vi "Check Data Size (excel).vi"(1 "error in (no error)":errorcluster, 2 "rect":T1, 3 "depth":u8, 4 "flattened image data":u8[](array[numeric])) -> (0 "error out":errorcluster)   [LabVIEW 2020, in "NI_ReportGenerationToolkit.lvlib"]
doc: "Checks the flattened data to see if the size of the data in bytes is what we expect it to be based on its bounds and depth."
uses:
  <vilib>/addons/_office/NI_ReportGenerationToolkit.lvlib
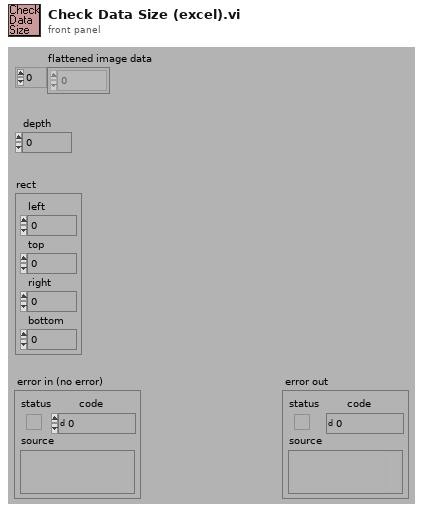
[diagram p1: front panel]
types:
  T1 = cluster{"left":i16, "top":i16, "right":i16, "bottom":i16}
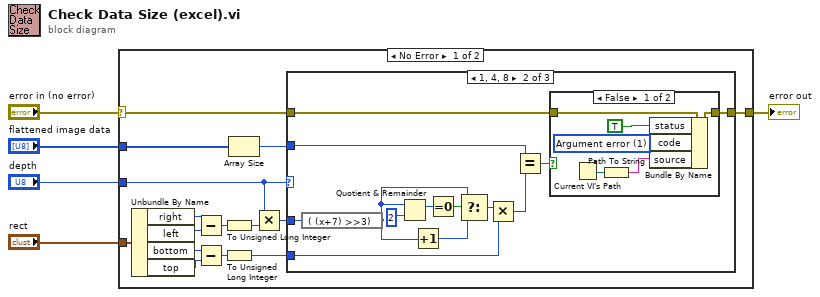
[diagram p0: block diagram]
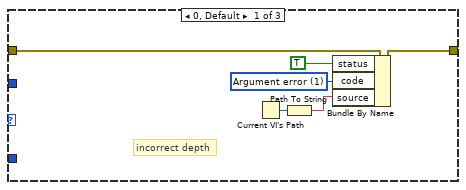
[diagram p2: hidden frame]
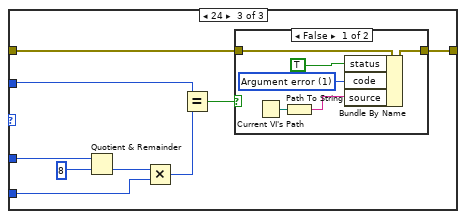
[diagram p4: hidden frame]
diagram:
  n1 = case shown="No Error" "error in (no error)" {
    selector: "error in (no error)" -> [w6 w63]
    tunnel: "depth" -> [w17 _]
    tunnel: "rect" -> [w16 _]
    tunnel: [w10 w63] -> w3
    tunnel: "flattened image data" -> [w9 _]
    frame No Error {
      n2 = Unbundle By Name(w16) -> ("right"=w11:i16, "left"=w12:i16, "bottom"=w15:i16, "top"=w14:i16)
      n3 = Subtract(x=w11, y=w12) -> (x-y=w13:i16)
      n4 = Subtract(x=w15, y=w14) -> (x-y=w18:i16)
      n5 = To Unsigned Long Integer(number=w13) -> (unsigned 32bit integer=w8:u32)
      n6 = To Unsigned Long Integer(number=w18) -> (unsigned 32bit integer=w7:u32)
      n7 = Array Size(array=w9) -> (size(s)=w20:i32)
      n8 = Multiply(x=w17, y=w8) -> (x*y=w19:u32)
      n9 = case shown="1, 4, 8" w17 {
        tunnel: w6 -> [w22 w33 w53]
        tunnel: [w21 w37 w52] -> w10
        tunnel: w7 -> [_ w36 w48]
        tunnel: w19 -> [_ w35 w51]
        tunnel: w20 -> [_ w34 w55]
        frame 0, Default {
          w25 = 1 items=["No error", "Argument error", "Memory is full", "Out of zone", "End of file", "File already open", "Generic file I/O error", "File not found", "File permission error", "Disk is full", "Duplicate path", "Too many files open", "System feature not enabled", "Resource file not found", "Cannot add resource", "Resource not found", "Image not found", "Image memory error", "Pen does not exist", "Config type invalid", "Config token not found", "Config parse error", "Config memory error", "Bad external code format", "Bad external code offset", "External code not present", "Null window", "Destroy window error", "Null menu", "Print aborted", "Bad print record", "Print driver error", "Windows error during printing", "Memory error during printing", "Print dialog error", "Generic print error", "Invalid device refnum", "Device not found", "Device parameter error", "Device unit error", "Cannot open device", "Device call aborted", "Generic error", "Cancelled by user", "Object ID too low", "Object ID too high", "Object not in heap", "Unknown heap", "Unknown object (invalid DefProc)", "Unknown object (DefProc not in table)", "Message out of range", "Invalid (null) method", "Unknown message", "Manager call not supported", "Bad address", "Network operation in progress", "Network operation timed out", "Connection is busy", "Network attribute not supported", "Network error", "Address in use", "System out of memory", "Connection aborted", "Connection refused", "Not connected", "Already connected", "Connection closed", "Initialization error (interapplication manager)", "Bad occurrence", "Wait on unbound occurrence handler", "Occurrence queue overflow", "Datalog type conflict", "Unused", "Unrecognized type (interapplication manager)", "Memory corrupt", "Failed to make temporary DLL", "Old CIN version", "Drag socket not found", "Failed to load drop-object", "Failed to register OLE object", "Failed to release OLE object", "Format specifier type mismatch", "Unknown format specifier", "Too few format specifiers", "Too many format specifiers", "Scan failed", "Newer CIN version", "Error converting to variant", "Runtime menu error", "Password tampered", "Variant attribute not found", "Incompatible variant data type", "Event data is not available", "Event Store is not present", "Occurrence is not found", "Event Queue is not created", "Event info is not available", "Refnum passed is NULL", "Error retrieving Class GUID", "Error retrieving CoClass GUID", "Error retrieving TypeLib GUID.", "Bad built application magic bytes.", "Specific driver is different from the specific driver associated with the Logical Name.", "There is no session opened to the class driver.", "Max Error", "MAX - Error with config objects", "MAX - Error loading configuration", "MAX - Group not supported"]
          # "incorrect depth"
          n10 = Current VI's Path() -> (path=w24:path)
          n11 = Path To String(path=w24) -> (string=w23:string)
          n12 = Bundle By Name(cluster=w22, "status"=TRUE, "code"=w25, "source"=w23) -> (w21:errorcluster)
        }
        frame 1, 4, 8 {
          n13 = expression code="(\t(x+7) >>3)"(w35) -> (w28:u32)
          n14 = Quotient & Remainder(x=w28, y=u32 2 ("x")) -> (x-y*floor(x/y)=w32:u32)  [unwired: 1 out]
          n15 = Increment(x=w28) -> (x+1=w31:u32)
          n16 = Equal To 0?(x=w32) -> (x = 0?=w30:bool)
          n17 = Select(t=w28, s=w30, f=w31) -> (s? t:f=w29:u32)
          n18 = Multiply(x=w29, y=w36) -> (x*y=w39:u32)
          n19 = Equal?(x=w34, y=w39) -> (x = y?=w38:bool)
          n20 = case shown="False" w38 {
            tunnel: w33 -> [w41 w46]
            tunnel: [w40 w46] -> w37
            frame False {
              w44 = 1 items=["No error", "Argument error", "Memory is full", "Out of zone", "End of file", "File already open", "Generic file I/O error", "File not found", "File permission error", "Disk is full", "Duplicate path", "Too many files open", "System feature not enabled", "Resource file not found", "Cannot add resource", "Resource not found", "Image not found", "Image memory error", "Pen does not exist", "Config type invalid", "Config token not found", "Config parse error", "Config memory error", "Bad external code format", "Bad external code offset", "External code not present", "Null window", "Destroy window error", "Null menu", "Print aborted", "Bad print record", "Print driver error", "Windows error during printing", "Memory error during printing", "Print dialog error", "Generic print error", "Invalid device refnum", "Device not found", "Device parameter error", "Device unit error", "Cannot open device", "Device call aborted", "Generic error", "Cancelled by user", "Object ID too low", "Object ID too high", "Object not in heap", "Unknown heap", "Unknown object (invalid DefProc)", "Unknown object (DefProc not in table)", "Message out of range", "Invalid (null) method", "Unknown message", "Manager call not supported", "Bad address", "Network operation in progress", "Network operation timed out", "Connection is busy", "Network attribute not supported", "Network error", "Address in use", "System out of memory", "Connection aborted", "Connection refused", "Not connected", "Already connected", "Connection closed", "Initialization error (interapplication manager)", "Bad occurrence", "Wait on unbound occurrence handler", "Occurrence queue overflow", "Datalog type conflict", "Unused", "Unrecognized type (interapplication manager)", "Memory corrupt", "Failed to make temporary DLL", "Old CIN version", "Drag socket not found", "Failed to load drop-object", "Failed to register OLE object", "Failed to release OLE object", "Format specifier type mismatch", "Unknown format specifier", "Too few format specifiers", "Too many format specifiers", "Scan failed", "Newer CIN version", "Error converting to variant", "Runtime menu error", "Password tampered", "Variant attribute not found", "Incompatible variant data type", "Event data is not available", "Event Store is not present", "Occurrence is not found", "Event Queue is not created", "Event info is not available", "Refnum passed is NULL", "Error retrieving Class GUID", "Error retrieving CoClass GUID", "Error retrieving TypeLib GUID.", "Bad built application magic bytes.", "Specific driver is different from the specific driver associated with the Logical Name.", "There is no session opened to the class driver.", "Max Error", "MAX - Error with config objects", "MAX - Error loading configuration", "MAX - Group not supported"]
              n21 = Current VI's Path() -> (path=w43:path)
              n22 = Path To String(path=w43) -> (string=w42:string)
              n23 = Bundle By Name(cluster=w41, "status"=TRUE, "code"=w44, "source"=w42) -> (w40:errorcluster)
            }
            frame True {
            }
          }
        }
        frame 24 {
          n24 = Quotient & Remainder(x=w51, y=u32 8) -> (floor(x/y)=w49:u32)  [unwired: 1 out]
          n25 = Multiply(x=w49, y=w48) -> (x*y=w47:u32)
          n26 = Equal?(x=w55, y=w47) -> (x = y?=w54:bool)
          n27 = case shown="False" w54 {
            tunnel: w53 -> [w57 w62]
            tunnel: [w56 w62] -> w52
            frame False {
              w60 = 1 items=["No error", "Argument error", "Memory is full", "Out of zone", "End of file", "File already open", "Generic file I/O error", "File not found", "File permission error", "Disk is full", "Duplicate path", "Too many files open", "System feature not enabled", "Resource file not found", "Cannot add resource", "Resource not found", "Image not found", "Image memory error", "Pen does not exist", "Config type invalid", "Config token not found", "Config parse error", "Config memory error", "Bad external code format", "Bad external code offset", "External code not present", "Null window", "Destroy window error", "Null menu", "Print aborted", "Bad print record", "Print driver error", "Windows error during printing", "Memory error during printing", "Print dialog error", "Generic print error", "Invalid device refnum", "Device not found", "Device parameter error", "Device unit error", "Cannot open device", "Device call aborted", "Generic error", "Cancelled by user", "Object ID too low", "Object ID too high", "Object not in heap", "Unknown heap", "Unknown object (invalid DefProc)", "Unknown object (DefProc not in table)", "Message out of range", "Invalid (null) method", "Unknown message", "Manager call not supported", "Bad address", "Network operation in progress", "Network operation timed out", "Connection is busy", "Network attribute not supported", "Network error", "Address in use", "System out of memory", "Connection aborted", "Connection refused", "Not connected", "Already connected", "Connection closed", "Initialization error (interapplication manager)", "Bad occurrence", "Wait on unbound occurrence handler", "Occurrence queue overflow", "Datalog type conflict", "Unused", "Unrecognized type (interapplication manager)", "Memory corrupt", "Failed to make temporary DLL", "Old CIN version", "Drag socket not found", "Failed to load drop-object", "Failed to register OLE object", "Failed to release OLE object", "Format specifier type mismatch", "Unknown format specifier", "Too few format specifiers", "Too many format specifiers", "Scan failed", "Newer CIN version", "Error converting to variant", "Runtime menu error", "Password tampered", "Variant attribute not found", "Incompatible variant data type", "Event data is not available", "Event Store is not present", "Occurrence is not found", "Event Queue is not created", "Event info is not available", "Refnum passed is NULL", "Error retrieving Class GUID", "Error retrieving CoClass GUID", "Error retrieving TypeLib GUID.", "Bad built application magic bytes.", "Specific driver is different from the specific driver associated with the Logical Name.", "There is no session opened to the class driver.", "Max Error", "MAX - Error with config objects", "MAX - Error loading configuration", "MAX - Group not supported"]
              n28 = Current VI's Path() -> (path=w59:path)
              n29 = Path To String(path=w59) -> (string=w58:string)
              n30 = Bundle By Name(cluster=w57, "status"=TRUE, "code"=w60, "source"=w58) -> (w56:errorcluster)
            }
            frame True {
            }
          }
        }
      }
    }
    frame Error {
    }
  }
  "error out" <- w3
